vi "Eval Multi-Variable Array.vi"(2 "error in (no error)":errorcluster, 3 "Variables":string[](array[string]), 4 "X Values":dbl[][](array[numeric]) format="%.2f", 5 "formula":string) -> (0 "error out":errorcluster, 1 "Y Values":dbl[](array[numeric]) format="%.2f")   [LabVIEW 2020, in "NI_Gmath.lvlib"]
doc: "Calculates the function values of a given function at an arbitrarily given set of n dimension points."
uses:
  NI_Gmath.lvlib
panel:
  # "Example:\n\n formula: x*sin(y)\n X Values: ((1.0,1.0,2.0),(2.2,3.14,6.28))  \n Variables: x and y"
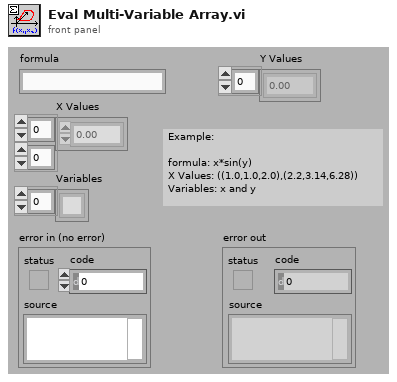
[diagram p1: front panel]
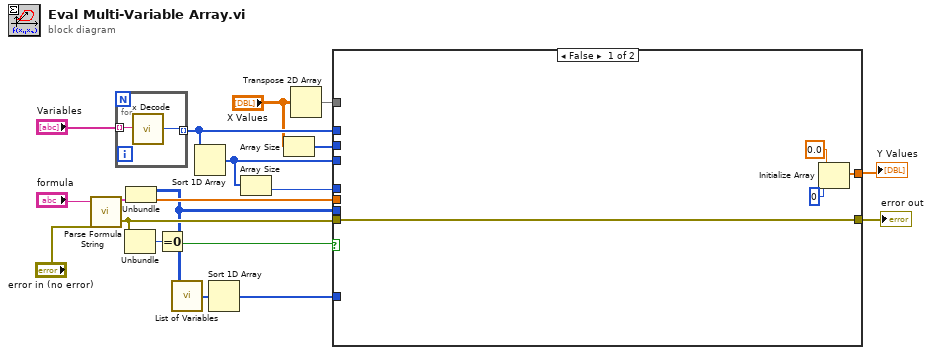
[diagram p0: block diagram]
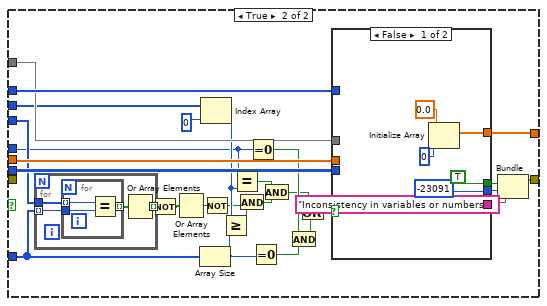
[diagram p2: hidden frame]
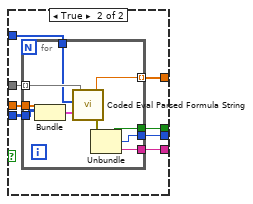
[diagram p3: hidden frame]
diagram:
  n1 = call "Parse Formula String.vi"("error in (no error)"="error in (no error)", "formula"="formula") -> ("error out"=w10:errorcluster, "Parsed Formula"=w5:cluster{"Table":i32[][], "Y Values":dbl[]})
  n2 = for {
    tunnel: "Variables" -> [w21] mode=indexing
    tunnel: [w20] -> w16 mode=indexing
    n3 = call "x Decode.vi"("x string"=w21) -> ("number"=w20:i32)  [unwired: 1 in, 1 out]
  }
  n4 = Unbundle(w10) -> ("code"=w9:i32)  [unwired: 2 out]
  n5 = Unbundle(w5) -> ("Table"=w3:i32[][], "Y Values"=w4:dbl[])
  n6 = Equal To 0?(x=w9) -> (x = 0?=w18:bool)
  n7 = call "List of Variables.vi"("Table"=w3) -> ("List of variables"=w15:i32[])
  n8 = Sort 1D Array(array=w16) -> (sorted array=w8:i32[])
  n9 = Sort 1D Array(array=w15) -> (sorted array=w6:i32[])
  n10 = Array Size(array=w8) -> (size(s)=w7:i32)
  n11 = Array Size(array="X Values") -> (size(s)=w12:i32[])
  n12 = Transpose 2D Array(2D array="X Values") -> (transposed array=w11:dbl[][])
  n13 = case shown="False" w18 {
    tunnel: [w22 w52] -> w14
    tunnel: w10 -> [w25 _]
    tunnel: w4 -> [_ w51]
    tunnel: w3 -> [_ w53]
    tunnel: w11 -> [_ w48]
    tunnel: w16 -> [_ w50]
    tunnel: w8 -> [_ w36]
    tunnel: w6 -> [_ w37]
    tunnel: w12 -> [_ w47]
    tunnel: [w25 w41] -> w1
    tunnel: w7 -> [_ w34]
    frame False {
      n14 = Initialize Array(0.0, 0) -> (w22:dbl[])
    }
    frame True {
      n15 = for {
        tunnel: w37 -> [w57] mode=indexing
        tunnel: w36 -> [w56]
        tunnel: [w54] -> w35 mode=indexing
        n16 = for {
          tunnel: w57 -> [w60]
          tunnel: w56 -> [w59] mode=indexing
          tunnel: [w58] -> w55 mode=indexing
          n17 = Equal?(x=w59, y=w60) -> (x = y?=w58:bool)
        }
        n18 = Or Array Elements(Boolean array=w55) -> (logical OR=w54:bool)
      }
      n19 = Not(x=w35) -> (.not. x?=w27:bool[])
      n20 = Or Array Elements(Boolean array=w27) -> (logical OR=w28:bool)
      n21 = Array Size(array=w37) -> (size(s)=w45:i32)
      n22 = Index Array(array=w47, index=0) -> (element=w40:i32)
      n23 = Not(x=w28) -> (.not. x?=w26:bool)
      n24 = Greater Or Equal?(x=w40, y=w45) -> (x >= y?=w49:bool)
      n25 = Equal?(x=w34, y=w40) -> (x = y?=w39:bool)
      n26 = And(x=w26, y=w49) -> (x .and. y?=w38:bool)
      n27 = Equal To 0?(x=w34) -> (x = 0?=w33:bool)
      n28 = Equal To 0?(x=w45) -> (x = 0?=w32:bool)
      n29 = And(x=w39, y=w38) -> (x .and. y?=w31:bool)
      n30 = And(x=w33, y=w32) -> (x .and. y?=w30:bool)
      n31 = Or(x=w31, y=w30) -> (x .or. y?=w29:bool)
      n32 = case shown="False" w29 {
        tunnel: w48 -> [_ w74]
        tunnel: [w61 w73] -> w52
        tunnel: w53 -> [_ w72]
        tunnel: w51 -> [_ w71]
        tunnel: w50 -> [_ w70]
        tunnel: [TRUE w69] -> w44
        tunnel: [-23091 w68] -> w43
        tunnel: ["Inconsistency in variables or numbers" w67] -> w42
        frame False {
          n33 = Initialize Array(0.0, 0) -> (w61:dbl[])
        }
        frame True {
          n34 = for {
            tunnel: w70 -> [w77]
            tunnel: w71 -> [w75]
            tunnel: w72 -> [w76]
            tunnel: [w84] -> w73 mode=indexing
            tunnel: w74 -> [w78] mode=indexing
            tunnel: [w82] -> w69
            tunnel: [w81] -> w68
            tunnel: [w80] -> w67
            n35 = Bundle("Table"=w76, "Y Values"=w75) -> (w79:cluster{"Table":i32[][], "Y Values":dbl[]})  [unwired: 1 in]
            n36 = call "Coded Eval Parsed Formula String.vi"("Parsed Formula"=w79, "Variables"=w77, "X Values"=w78) -> ("error out"=w83:errorcluster, "y value"=w84:dbl)  [unwired: 1 in]
            n37 = Unbundle(w83) -> ("status"=w82:bool, "code"=w81:i32, "source"=w80:string)
          }
        }
      }
      n38 = Bundle("status"=w44, "code"=w43, "source"=w42) -> (w41:errorcluster)  [unwired: 1 in]
    }
  }
  "Y Values" <- w14
  "error out" <- w1
